vi "Send Cmd.vi"(8 "error in (no error)":errorcluster, 10 "Command":string, 11 "Reload-pro in":refnum<class "Reload-pro.lvclass">) -> (0 "error out":errorcluster, 2 "Response":string, 3 "Reload-pro out":refnum<class "Reload-pro.lvclass">)   [LabVIEW 2013, in "Reload-pro.lvclass"]
uses:
  Reload-pro.lvclass
  Reload-pro.lvclass/Reload-pro.ctl
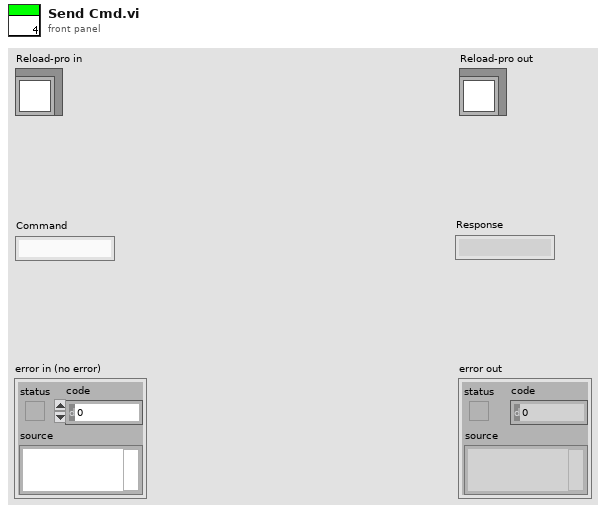
[diagram p1: front panel]
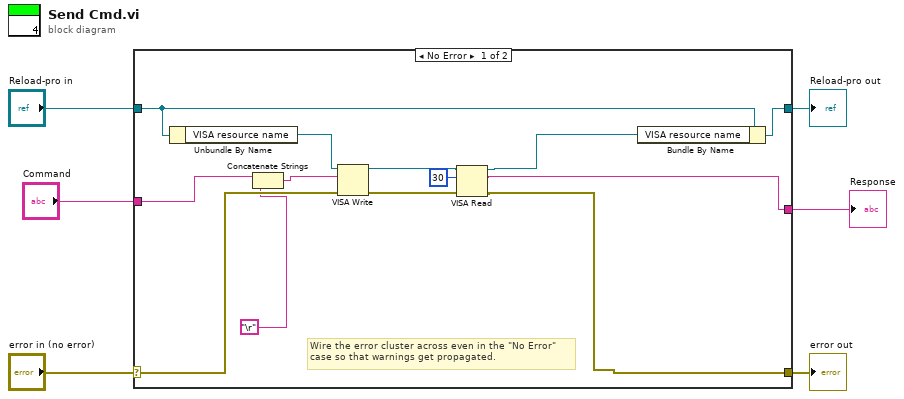
[diagram p0: block diagram]
diagram:
  n1 = case shown="No Error" "error in (no error)" {
    selector: "error in (no error)" -> [w16 w21]
    tunnel: [w8 w21] -> w5
    tunnel: [w19 w20] -> w3
    tunnel: "Reload-pro in" -> [w18 w20]
    tunnel: [w7 _] -> w2
    tunnel: "Command" -> [w15 _]
    frame No Error {
      # "Wire the error cluster across even in the \"No Error\"\ncase so that warnings get propagated."
      n2 = Unbundle By Name(w18) -> ("VISA resource name"=w17:refnum<visa-resource-name>)
      n3 = Concatenate Strings(w15, "\r") -> (w13:string)
      n4 = VISA Write(VISA resource name=w17, write buffer=w13, error in (no error)=w16) -> (VISA resource name out=w12:refnum<visa-resource-name>, error out=w11:errorcluster)  [unwired: 1 out]
      n5 = VISA Read(VISA resource name=w12, byte count=u32 30, error in (no error)=w11) -> (VISA resource name out=w9:refnum<visa-resource-name>, read buffer=w7:string, error out=w8:errorcluster)  [unwired: 1 out]
      n6 = Bundle By Name(cluster=w18, "VISA resource name"=w9) -> (w19:refnum<class "Reload-pro.lvclass">)
    }
    frame Error {
    }
  }
  "error out" <- w5
  "Reload-pro out" <- w3
  "Response" <- w2
